vi "RsRp计算.vi"(5 "I":dbl[](array[numeric]), 7 "A":dbl[](array[numeric]), 9 "压力点个数":dbl=3.0, 10 "检定次数":dbl=1.0, 11 "数据":dbl[][](array[numeric])) -> (1 "Rs 2":dbl[](array[numeric]), 2 "Rs":dbl[](array[numeric]), 3 "Rp":dbl[](array[numeric]))   [LabVIEW 2017]
uses:
  <vilib>/Analysis/Matrix/Datatypes/RealMatrix.ctl
  793ac652-eb95-4cdd-88e1-b3e4c67dd276.vi
  348b27d3-cf50-41c3-8648-c04ad73e2cb6.vi
  <vilib>/Array/Sort 2D Array - Pop Stack.vi
  <vilib>/Array/Sort 2D Array - Push Stack.vi
  <vilib>/Analysis/Matrix/NI_Matrix.lvlib
panel:
  in  "退出":bool
  out "70反":dbl[][](array[numeric])
  out "70正":dbl[][](array[numeric])
  out "-40反":dbl[][](array[numeric])
  out "-40正":dbl[][](array[numeric])
  out "70反平均":dbl[][](array[numeric])
  out "70正平均":dbl[][](array[numeric])
  out "-40反平均":dbl[][](array[numeric])
  out "-40正平均":dbl[][](array[numeric])
  out "x/y 2":T1 caption="x/y"
  out "x/y":T1
  out "-40满量程桥压":dbl[](array[numeric])
  out "-40常压桥压":dbl[](array[numeric])
  out "-40常压输出":dbl[](array[numeric])
  out "-40满量程输出":dbl[](array[numeric])
  out "70满量程桥压":dbl[](array[numeric])
  out "70常压桥压":dbl[](array[numeric])
  out "70常压输出":dbl[](array[numeric])
  out "70满量程输出":dbl[](array[numeric])
  # "补偿电阻计算"
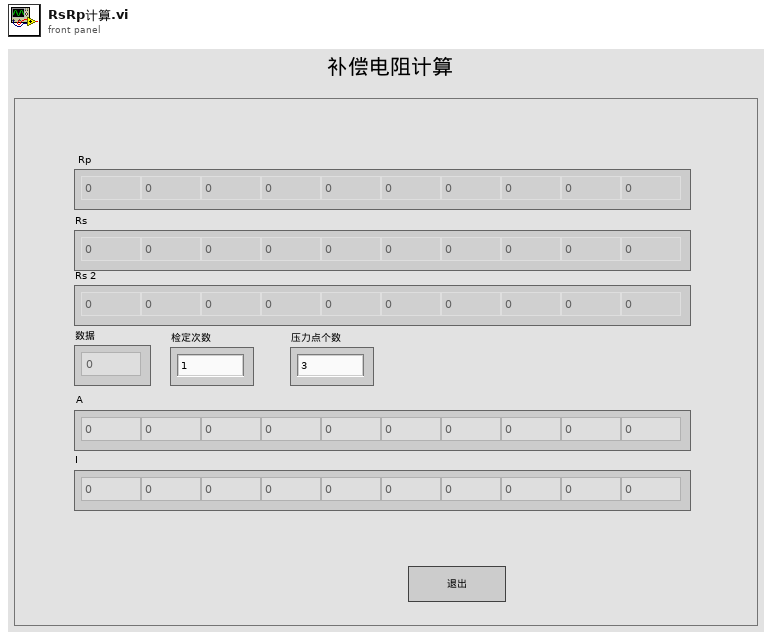
[diagram p1: front panel]
types:
  T1 = typedef "NI_Matrix.lvlib/RealMatrix.ctl" = dbl[][]
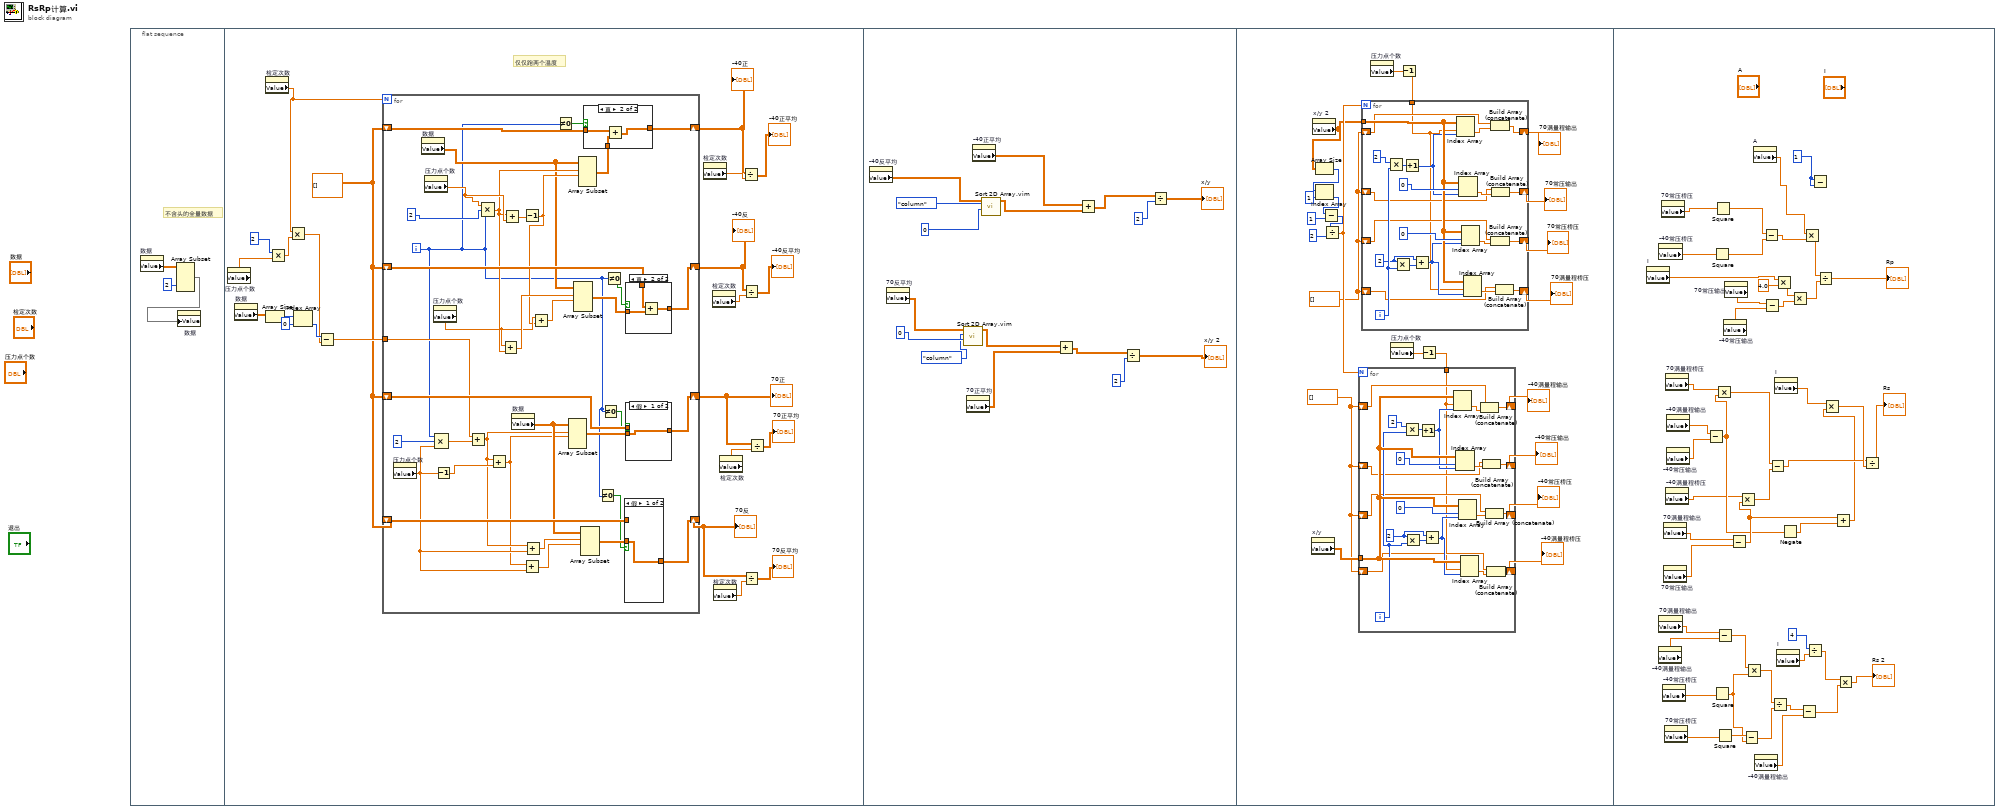
[diagram p0: block diagram]
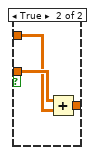
[diagram p2: hidden frame]
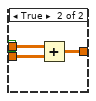
[diagram p3: hidden frame]
diagram:
  n1 = flat-sequence {
    frame #0 {
      # "不含头的全量数据"
      n2 = property on="数据" class="Arr (严格)"() -> ("Value"=w3:dbl[][])  [unwired: 2 in, 2 out]
      n3 = Array Subset(array=w3, index (col)=2 ("索引")) -> (w1:dbl[][])  [unwired: 3 in]
      n4 = property on="数据" class="Arr (严格)"("Value"=w1) -> ()  [unwired: 2 in, 2 out]
    }
    frame #1 {
      w4 = dbl[][] []
      # "仅仅跑两个温度"
      n5 = property on="压力点个数" class="DigNum (严格)"() -> ("Value"=w10:dbl)  [unwired: 2 in, 2 out]
      n6 = property on="数据" class="Arr (严格)"() -> ("Value"=w14:dbl[][])  [unwired: 2 in, 2 out]
      n7 = property on="检定次数" class="DigNum (严格)"() -> ("Value"=w8:dbl)  [unwired: 2 in, 2 out]
      n8 = Array Size(array=w14) -> (size(s)=w13:i32[])
      n9 = Multiply(x=2, y=w10) -> (x*y=w9:dbl)
      n10 = Multiply(x=w8, y=w9) -> (x*y=w6:dbl)
      n11 = Index Array(array=w13, index=0 ("索引")) -> (element=w7:i32)
      n12 = Subtract(x=w7, y=w6) -> (x-y=w5:dbl)
      n13 = for {
        N: w8 -> [_]
        shift-right: [w50] -> w21
        shift-left: w4 -> [w60]
        shift-right: [w49] -> w15
        shift-left: w4 -> [w58]
        shift-right: [w48] -> w16
        shift-left: w4 -> [w56]
        shift-right: [w52] -> w25
        shift-left: w4 -> [w51]
        tunnel: w5 -> [w40]
        i -> [w28]
        n14 = property on="压力点个数" class="DigNum (严格)"() -> ("Value"=w37:dbl)  [unwired: 2 in, 2 out]
        n15 = property on="数据" class="Arr (严格)"() -> ("Value"=w32:dbl[][])  [unwired: 2 in, 2 out]
        n16 = property on="压力点个数" class="DigNum (严格)"() -> ("Value"=w55:dbl)  [unwired: 2 in, 2 out]
        n17 = property on="压力点个数" class="DigNum (严格)"() -> ("Value"=w44:dbl)  [unwired: 2 in, 2 out]
        n18 = Compound Arithmetic op=MULTIPLY(w28, 2, w37) -> (w41:dbl)
        n19 = Decrement(x=w37) -> (x-1=w39:dbl)
        n20 = Add(x=w40, y=w41) -> (x+y=w36:dbl)
        n21 = Compound Arithmetic op=MULTIPLY(w55, 2, w28) -> (w46:dbl)
        n22 = Add(x=w36, y=w39) -> (x+y=w35:dbl)
        n23 = Add(x=w44, y=w46) -> (x+y=w47:dbl)
        n24 = Add(x=w46, y=w55) -> (x+y=w62:dbl)
        n25 = property on="数据" class="Arr (严格)"() -> ("Value"=w38:dbl[][])  [unwired: 2 in, 2 out]
        n26 = Add(x=w35, y=w37) -> (x+y=w33:dbl)
        n27 = Decrement(x=w62) -> (x-1=w43:dbl)
        n28 = Add(x=w36, y=w37) -> (x+y=w34:dbl)
        n29 = Add(x=w44, y=w43) -> (x+y=w45:dbl)
        n30 = Not Equal To 0?(x=w28) -> (x != 0?=w31:bool)
        n31 = Array Subset(array=w38, index (row)=w36, length (row)=w35) -> (w59:dbl[][])  [unwired: 2 in]
        n32 = Array Subset(array=w32, index (row)=w47, length (row)=w45) -> (w61:dbl[][])  [unwired: 2 in]
        n33 = Array Subset(array=w32, index (row)=w46, length (row)=w43) -> (w53:dbl[][])  [unwired: 2 in]
        n34 = Array Subset(array=w38, index (row)=w34, length (row)=w33) -> (w57:dbl[][])  [unwired: 2 in]
        n35 = case shown="真" w31 {
          tunnel: w53 -> [w75 w78]
          tunnel: [w75 w77] -> w52
          tunnel: w51 -> [_ w76]
          frame False {
          }
          frame True {
            n36 = Add ("Add.vi")(x=w76, y=w78) -> (x+y=w77:dbl[][])
          }
        }
        n37 = Not Equal To 0?(x=w28) -> (x != 0?=w27:bool)
        n38 = Not Equal To 0?(x=w28) -> (x != 0?=w29:bool)
        n39 = Not Equal To 0?(x=w28) -> (x != 0?=w30:bool)
        n40 = case shown="假" w27 {
          tunnel: w57 -> [w63 w66]
          tunnel: w56 -> [_ w65]
          tunnel: [w63 w64] -> w48
          frame False {
          }
          frame True {
            n41 = Add ("Add.vi")(x=w66, y=w65) -> (x+y=w64:dbl[][])
          }
        }
        n42 = case shown="真" w30 {
          tunnel: w61 -> [w71 w74]
          tunnel: w60 -> [_ w73]
          tunnel: [w71 w72] -> w50
          frame False {
          }
          frame True {
            n43 = Add ("Add.vi")(x=w73, y=w74) -> (x+y=w72:dbl[][])
          }
        }
        n44 = case shown="假" w29 {
          tunnel: w59 -> [w67 w70]
          tunnel: w58 -> [_ w69]
          tunnel: [w67 w68] -> w49
          frame False {
          }
          frame True {
            n45 = Add(x=w69, y=w70) -> (x+y=w68:dbl[][])
          }
        }
      }
      "-40正" <- w25
      "-40反" <- w21
      "70正" <- w15
      "70反" <- w16
      n46 = property on="检定次数" class="DigNum (严格)"() -> ("Value"=w26:dbl)  [unwired: 2 in, 2 out]
      n47 = property on="检定次数" class="DigNum (严格)"() -> ("Value"=w23:dbl)  [unwired: 2 in, 2 out]
      n48 = property on="检定次数" class="DigNum (严格)"() -> ("Value"=w18:dbl)  [unwired: 2 in, 2 out]
      n49 = property on="检定次数" class="DigNum (严格)"() -> ("Value"=w19:dbl)  [unwired: 2 in, 2 out]
      n50 = Divide(x=w25, y=w26) -> (x/y=→"-40正平均":dbl[][])
      n51 = Divide(x=w21, y=w23) -> (x/y=→"-40反平均":dbl[][])
      n52 = Divide(x=w16, y=w18) -> (x/y=→"70反平均":dbl[][])
      n53 = Divide(x=w15, y=w19) -> (x/y=→"70正平均":dbl[][])
    }
    frame #2 {
      n54 = property on="-40反平均" class="Arr (严格)"() -> ("Value"=w92:dbl[][])  [unwired: 2 in, 2 out]
      n55 = property on="70反平均" class="Arr (严格)"() -> ("Value"=w94:dbl[][])  [unwired: 2 in, 2 out]
      n56 = call "Sort 2D Array.vim"("index"=0, "dimension to index (column)"=enum16{"column", "row"}."column", "2D array"=w94) -> ("sorted 2D array"=w90:dbl[][])  [unwired: 7 in, 1 out]
      n57 = property on="70正平均" class="Arr (严格)"() -> ("Value"=w93:dbl[][])  [unwired: 2 in, 2 out]
      n58 = property on="-40正平均" class="Arr (严格)"() -> ("Value"=w91:dbl[][])  [unwired: 2 in, 2 out]
      n59 = call "Sort 2D Array.vim"("index"=0, "dimension to index (column)"=enum16{"column", "row"}."column", "2D array"=w92) -> ("sorted 2D array"=w89:dbl[][])  [unwired: 7 in, 1 out]
      n60 = Add ("Add.vi")(x=w90, y=w93) -> (x+y=w88:dbl[][])
      n61 = Add ("Add.vi")(x=w91, y=w89) -> (x+y=w87:dbl[][])
      n62 = Divide(x=w88, y=2) -> (x/y=→"x/y 2":dbl[][])
      n63 = Divide(x=w87, y=2) -> (x/y=→"x/y":dbl[][])
    }
    frame #3 {
      w99 = dbl[] []
      w100 = dbl[] []
      n64 = property on="x/y" class="Arr (严格)"() -> ("Value"=w112:T1)  [unwired: 2 in, 2 out]
      n65 = property on="x/y 2" class="Arr (严格)"() -> ("Value"=w113:T1)  [unwired: 2 in, 2 out]
      n66 = Array Size(array=w113) -> (size(s)=w114:i32[])
      n67 = Index Array(array=w114, index=1 ("索引")) -> (element=w115:i32)
      n68 = Subtract(x=w115, y=1) -> (x-y=w116:i32)
      n69 = Divide(x=w116, y=2) -> (x/y=w117:dbl)
      n70 = property on="压力点个数" class="DigNum (严格)"() -> ("Value"=w98:dbl)  [unwired: 2 in, 2 out]
      n71 = property on="压力点个数" class="DigNum (严格)"() -> ("Value"=w96:dbl)  [unwired: 2 in, 2 out]
      n72 = Decrement(x=w98) -> (x-1=w97:dbl)
      n73 = for {
        N: w117 -> [_]
        tunnel: w113 -> [w161]
        shift-right: [w152] -> w104
        shift-left: w99 -> [w151]
        shift-right: [w149] -> w105
        shift-left: w99 -> [w148]
        shift-right: [w146] -> w106
        shift-left: w99 -> [w145]
        shift-right: [w143] -> w107
        shift-left: w99 -> [w142]
        tunnel: w97 -> [w141]
        i -> [w157]
        w155 = 2
        n74 = Multiply(x=2, y=w157) -> (x*y=w160:i32)
        n75 = Multiply(x=w155, y=w157) -> (x*y=w156:i32)
        n76 = Increment(x=w160) -> (x+1=w159:i32)
        n77 = Add(x=w155, y=w156) -> (x+y=w154:i32)
        n78 = Index Array(array=w161, index (row)=w141, index (col)=w159) -> (element=w153:dbl)
        n79 = Index Array(array=w161, index (row)=0, index (col)=w159) -> (element=w150:dbl)
        n80 = Index Array(array=w161, index (row)=0 ("索引 (行)"), index (col)=w154) -> (element=w147:dbl)
        n81 = Index Array(array=w161, index (row)=w141, index (col)=w154) -> (element=w144:dbl)
        n82 = Build Array (concatenate)(w151, w153) -> (w152:dbl[])
        n83 = Build Array (concatenate)(w145, w147) -> (w146:dbl[])
        n84 = Build Array (concatenate)(w148, w150) -> (w149:dbl[])
        n85 = Build Array (concatenate)(w142, w144) -> (w143:dbl[])
      }
      "70满量程输出" <- w104
      "70常压输出" <- w105
      "70常压桥压" <- w106
      "70满量程桥压" <- w107
      n86 = Decrement(x=w96) -> (x-1=w95:dbl)
      n87 = for {
        N: w117 -> [_]
        tunnel: w112 -> [w138]
        shift-right: [w129] -> w108
        shift-left: w100 -> [w128]
        shift-right: [w126] -> w109
        shift-left: w100 -> [w125]
        shift-right: [w123] -> w110
        shift-left: w100 -> [w122]
        shift-right: [w121] -> w111
        shift-left: w100 -> [w119]
        tunnel: w95 -> [w118]
        i -> [w131]
        w133 = 2
        n88 = Multiply(x=2, y=w131) -> (x*y=w137:i32)
        n89 = Multiply(x=w133, y=w131) -> (x*y=w134:i32)
        n90 = Increment(x=w137) -> (x+1=w135:i32)
        n91 = Add(x=w133, y=w134) -> (x+y=w132:i32)
        n92 = Index Array(array=w138, index (row)=w118, index (col)=w135) -> (element=w130:dbl)
        n93 = Index Array(array=w138, index (row)=0, index (col)=w135) -> (element=w127:dbl)
        n94 = Index Array(array=w138, index (row)=0 ("索引 (行)"), index (col)=w132) -> (element=w124:dbl)
        n95 = Index Array(array=w138, index (row)=w118, index (col)=w132) -> (element=w120:dbl)
        n96 = Build Array (concatenate)(w128, w130) -> (w129:dbl[])
        n97 = Build Array (concatenate)(w125, w127) -> (w126:dbl[])
        n98 = Build Array (concatenate)(w122, w124) -> (w123:dbl[])
        n99 = Build Array (concatenate)(w119, w120) -> (w121:dbl[])
      }
      "-40满量程输出" <- w108
      "-40常压输出" <- w109
      "-40常压桥压" <- w110
      "-40满量程桥压" <- w111
    }
    frame #4 {
      w180 = 1
      n100 = property on="I" class="Arr (严格)"() -> ("Value"=w211:dbl[])  [unwired: 2 in, 2 out]
      n101 = property on="-40满量程输出" class="Arr (严格)"() -> ("Value"=w176:dbl[])  [unwired: 2 in, 2 out]
      n102 = property on="-40常压桥压" class="Arr (严格)"() -> ("Value"=w184:dbl[])  [unwired: 2 in, 2 out]
      n103 = property on="70满量程输出" class="Arr (严格)"() -> ("Value"=w177:dbl[])  [unwired: 2 in, 2 out]
      n104 = property on="70常压桥压" class="Arr (严格)"() -> ("Value"=w183:dbl[])  [unwired: 2 in, 2 out]
      n105 = property on="-40常压桥压" class="Arr (严格)"() -> ("Value"=w175:dbl[])  [unwired: 2 in, 2 out]
      n106 = property on="70满量程输出" class="Arr (严格)"() -> ("Value"=w209:dbl[])  [unwired: 2 in, 2 out]
      n107 = property on="70常压输出" class="Arr (严格)"() -> ("Value"=w202:dbl[])  [unwired: 2 in, 2 out]
      n108 = property on="70常压桥压" class="Arr (严格)"() -> ("Value"=w173:dbl[])  [unwired: 2 in, 2 out]
      n109 = property on="70满量程桥压" class="Arr (严格)"() -> ("Value"=w195:dbl[])  [unwired: 2 in, 2 out]
      n110 = property on="-40满量程桥压" class="Arr (严格)"() -> ("Value"=w197:dbl[])  [unwired: 2 in, 2 out]
      n111 = property on="-40满量程输出" class="Arr (严格)"() -> ("Value"=w196:dbl[])  [unwired: 2 in, 2 out]
      n112 = property on="-40常压输出" class="Arr (严格)"() -> ("Value"=w203:dbl[])  [unwired: 2 in, 2 out]
      n113 = Subtract(x=w196, y=w203) -> (x-y=w201:dbl[])
      n114 = Square(x=w184) -> (x^2=w186:dbl[])
      n115 = Square(x=w175) -> (x^2=w171:dbl[])
      n116 = Square(x=w183) -> (x^2=w185:dbl[])
      n117 = Multiply(x=w195, y=w201) -> (x*y=w198:dbl[])
      n118 = Subtract(x=w177, y=w176) -> (x-y=w174:dbl[])
      n119 = Square(x=w173) -> (x^2=w172:dbl[])
      n120 = property on="-40常压输出" class="Arr (严格)"() -> ("Value"=w189:dbl[])  [unwired: 2 in, 2 out]
      n121 = property on="70常压输出" class="Arr (严格)"() -> ("Value"=w190:dbl[])  [unwired: 2 in, 2 out]
      n122 = Subtract(x=w209, y=w202) -> (x-y=w210:dbl[])
      n123 = Multiply(x=w197, y=w210) -> (x*y=w199:dbl[])
      n124 = Subtract(x=w172, y=w171) -> (x-y=w169:dbl[])
      n125 = Multiply(x=w174, y=w171) -> (x*y=w170:dbl[])
      n126 = property on="A" class="Arr (严格)"() -> ("Value"=w181:dbl[])  [unwired: 2 in, 2 out]
      n127 = property on="-40满量程输出" class="Arr (严格)"() -> ("Value"=w167:dbl[])  [unwired: 2 in, 2 out]
      n128 = Subtract(x=w185, y=w186) -> (x-y=w187:dbl[])
      n129 = Subtract(x=w190, y=w189) -> (x-y=w188:dbl[])
      n130 = Subtract(x=w198, y=w199) -> (x-y=w206:dbl[])
      n131 = Divide(x=w170, y=w169) -> (x/y=w168:dbl[])
      n132 = property on="I" class="Arr (严格)"() -> ("Value"=w200:dbl[])  [unwired: 2 in, 2 out]
      n133 = Multiply(x=w211, y=4.0) -> (x*y=w194:dbl[])
      n134 = property on="I" class="Arr (严格)"() -> ("Value"=w179:dbl[])  [unwired: 2 in, 2 out]
      n135 = Negate(x=w201) -> (-x=w204:dbl[])
      n136 = Multiply(x=w194, y=w188) -> (x*y=w191:dbl[])
      n137 = Subtract(x=w168, y=w167) -> (x-y=w165:dbl[])
      n138 = Multiply(x=w181, y=w187) -> (x*y=w192:dbl[])
      n139 = Divide(x=4, y=w179) -> (x/y=w166:dbl[])
      n140 = Subtract(x=w180, y=w180) -> ()  [unwired: 1 out]
      n141 = Divide(x=w192, y=w191) -> (x/y=→"Rp":dbl[])
      n142 = Add(x=w210, y=w204) -> (x+y=w205:dbl[])
      n143 = Multiply(x=w200, y=w205) -> (x*y=w207:dbl[])
      n144 = Multiply(x=w166, y=w165) -> (x*y=→"Rs 2":dbl[])
      n145 = Divide(x=w206, y=w207) -> (x/y=→"Rs":dbl[])
    }
  }
